vi "Destroy Request Events.vi"(8 "error in":errorcluster) -> (0 "error out":errorcluster)   [LabVIEW 2020, in "Manejador archivo.lvlib"]
doc: "Destroy the requests user events, even if there is an incoming error.\n\n<b>NOTE</b>: The contents of this VI are automatically generated and modified by the <b>Tools > DQMH Consortium > DQMH</b> utilities. Consider using those utilities instead of making your own modifications to this VI.\n_____\nBased on DQMH Dev Tools: Project Template 7.1.0.1490."
uses:
  Manejador archivo.lvlib
panel:
  # "NOTE: The contents of this VI are automatically generated and modified by the Tools > DQMH Consortium > DQMH utilities. Consider using those utilities instead of making your own modifications to this VI."
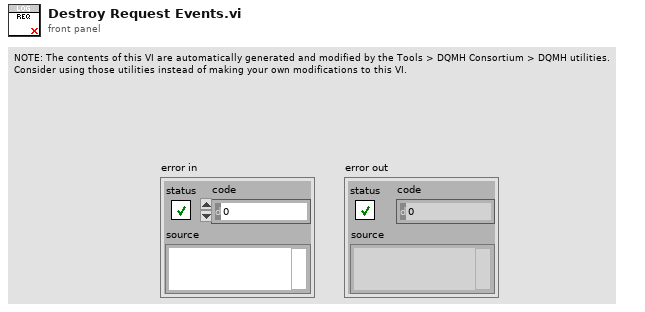
[diagram p1: front panel]
types:
  T1 = typedef "Manejador archivo.lvlib/Request Events--cluster.ctl" = cluster{"Stop Module":refnum<user-event>, "Show Panel":refnum<user-event>, "Hide Panel":refnum<user-event>, "Get Module Execution Status":refnum<user-event>, "Show Diagram":refnum<user-event>, "Set Column Headers":refnum<user-event>, "View File":refnum<user-event>, "Set File Path":refnum<user-event>, "Set File Settings":refnum<user-event>, "Log Data":refnum<user-event>, "Set File Format":refnum<user-event>, "Close File":refnum<user-event>, "Get Number of Columns":refnum<user-event>}
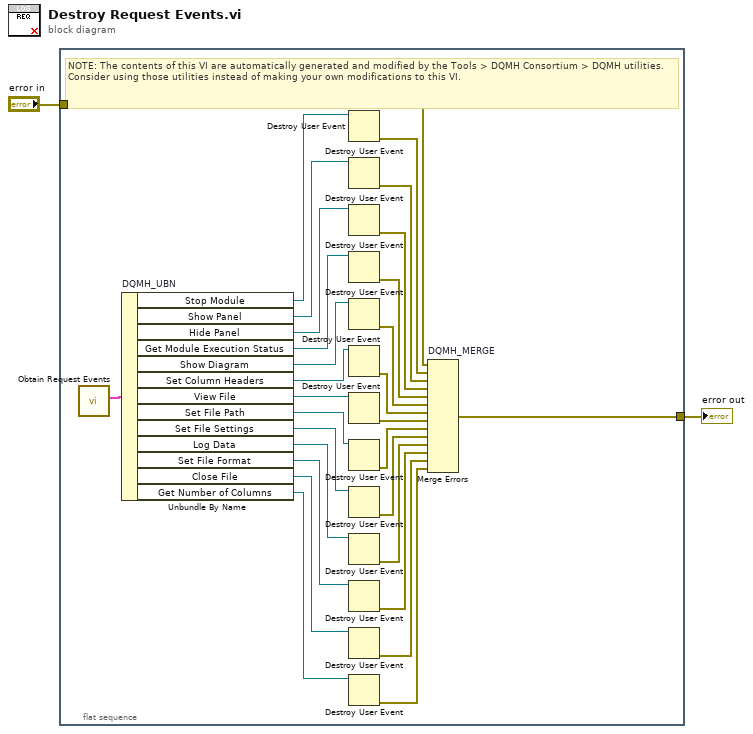
[diagram p0: block diagram]
diagram:
  n1 = flat-sequence {
    tunnel: [w30] -> w2
    tunnel: "error in" -> [w23]
    frame #0 {
      # "NOTE: The contents of this VI are automatically generated and modified by the Tools > DQMH Consortium > DQMH utilities. Consider using those utilities instead of making your own modifications to this VI."
      n2 = call "Obtain Request Events.vi"() -> ("Manejador archivo Request Events"=w29:T1)  [unwired: 10 in, 1 out]
      n3 = Unbundle By Name "DQMH_UBN"(w29) -> ("Stop Module"=w28:refnum<user-event>, "Show Panel"=w25:refnum<user-event>, "Hide Panel"=w24:refnum<user-event>, "Get Module Execution Status"=w21:refnum<user-event>, "Show Diagram"=w19:refnum<user-event>, "Set Column Headers"=w17:refnum<user-event>, "View File"=w15:refnum<user-event>, "Set File Path"=w13:refnum<user-event>, "Set File Settings"=w11:refnum<user-event>, "Log Data"=w9:refnum<user-event>, "Set File Format"=w7:refnum<user-event>, "Close File"=w5:refnum<user-event>, "Get Number of Columns"=w3:refnum<user-event>)
      n4 = Destroy User Event(user event=w28) -> (error out=w31:errorcluster)  [unwired: 1 in]
      n5 = Destroy User Event(user event=w25) -> (error out=w27:errorcluster)  [unwired: 1 in]
      n6 = Destroy User Event(user event=w24) -> (error out=w26:errorcluster)  [unwired: 1 in]
      n7 = Destroy User Event(user event=w21) -> (error out=w22:errorcluster)  [unwired: 1 in]
      n8 = Destroy User Event(user event=w19) -> (error out=w20:errorcluster)  [unwired: 1 in]
      n9 = Destroy User Event(user event=w17) -> (error out=w18:errorcluster)  [unwired: 1 in]
      n10 = Destroy User Event(user event=w15) -> (error out=w16:errorcluster)  [unwired: 1 in]
      n11 = Destroy User Event(user event=w13) -> (error out=w14:errorcluster)  [unwired: 1 in]
      n12 = Destroy User Event(user event=w11) -> (error out=w12:errorcluster)  [unwired: 1 in]
      n13 = Destroy User Event(user event=w9) -> (error out=w10:errorcluster)  [unwired: 1 in]
      n14 = Destroy User Event(user event=w7) -> (error out=w8:errorcluster)  [unwired: 1 in]
      n15 = Destroy User Event(user event=w5) -> (error out=w6:errorcluster)  [unwired: 1 in]
      n16 = Destroy User Event(user event=w3) -> (error out=w4:errorcluster)  [unwired: 1 in]
      n17 = Merge Errors "DQMH_MERGE"(w23, w31, w27, w26, w22, w20, w18, w16, w14, w12, w10, w8, w6, w4) -> (w30:errorcluster)
    }
  }
  "error out" <- w2
